vi "Process.vi"(8 "error in":errorcluster, 11 "Plugin in":refnum<class "Spectrogram.lvclass">) -> (0 "error out":errorcluster, 3 "Plugin out":refnum<class "Spectrogram.lvclass">)   [LabVIEW 2023, in "Spectrogram.lvlib" / "Spectrogram.lvclass"]
uses:
  Spectrogram.lvclass
  Spectrogram.lvclass/Spectrogram.ctl
  <vilib>/FlexLogger/SDK/PluginSDK.lvlibp/PEFClasses/SDK/Plugin/Plugin.lvclass
  C:/Program Files/National Instruments/LabVIEW 2023/vi.lib/FlexLogger/SDK/PluginSDK.lvlibp/PEFClasses/SDK/Plugin/Plugin.lvclass
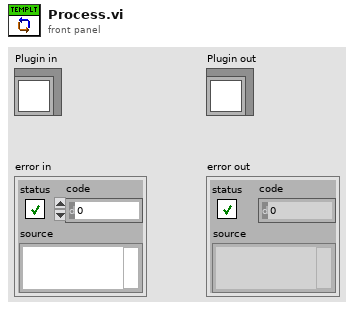
[diagram p1: front panel]
types:
  T1 = typedef "Spectrogram.lvlib/Spectrogram.lvclass/Spectrogram Data.ctl" = cluster{"First Time":bool, "Show Spectrogram Window":bool, "Show Spectrogram Window Button Clicked":bool, "Extension":u16, "Time steps":i32, "Frequency bins":i32, "Type":i32, "Length":i32, "Color Table":u16, "Spectrogram VI Ref":refnum<vi>}
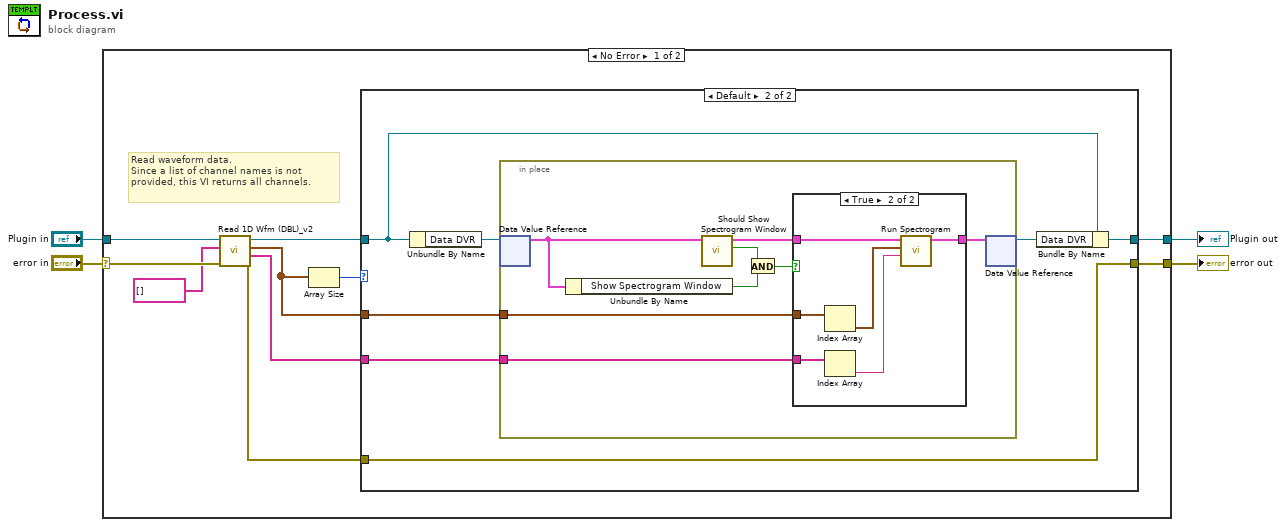
[diagram p0: block diagram]
diagram:
  n1 = case shown="No Error" "error in" {
    selector: "error in" -> [w13 w39]
    tunnel: [w11 w40] -> w1
    tunnel: "Plugin in" -> [w14 w40]
    tunnel: [w12 w39] -> w2
    frame No Error {
      # "Read waveform data.\nSince a list of channel names is not provided, this VI returns all channels."
      n2 = call <vilib>:"Read 1D Wfm (DBL)_v2.vi"("error in (no error)"=w13, "Unique Identifers (empty = all)"=string[] [] ("Unique Channel Identifers (empty = all)"), "Plugin in"=w14) -> ("error out"=w7:errorcluster, "Stream Names"=w5:string[], "Data"=w10:waveform(dbl)[], "Plugin out"=w8:refnum<class "Spectrogram.lvclass">)  [unwired: 5 in]
      n3 = Array Size(array=w10) -> (size(s)=w9:i32)
      n4 = case shown="Default" w9 {
        tunnel: w10 -> [_ w23]
        tunnel: [w15 w22] -> w12
        tunnel: [w16 w17] -> w11
        tunnel: w8 -> [w16 w18]
        tunnel: w7 -> [w15 w22]
        tunnel: w5 -> [_ w21]
        frame 0 {
          # "No channels sending data to the plugin"
        }
        frame Default {
          n5 = Unbundle By Name(w18) -> ("Data DVR"=w20:refnum<data-value>)
          n6 = in-place {
            in-place-border: w23 -> [w31]
            in-place-border: w21 -> [w28]
            n7 = in-place-dvr #1(w20) -> (w25:T1)  [unwired: 1 out]
            n8 = Unbundle By Name(w25) -> ("Show Spectrogram Window"=w30:bool)
            n9 = call "Should Show Spectrogram Window.vi"("Data in"=w25) -> ("Show Window"=w27:bool, "Data out"=w26:T1)  [unwired: 9 in]
            n10 = And(x=w27, y=w30) -> (x .and. y?=w29:bool)
            n11 = case shown="True" w29 {
              tunnel: w31 -> [_ w38]
              tunnel: w26 -> [w32 w36]
              tunnel: [w32 w35] -> w24
              tunnel: w28 -> [_ w37]
              frame False {
              }
              frame True {
                n12 = Index Array(array=w38) -> (element=w34:waveform(dbl))  [unwired: 1 in]
                n13 = Index Array(array=w37) -> (element=w33:string)  [unwired: 1 in]
                n14 = call "Run Spectrogram.vi"("Channel Name"=w33, "Signal"=w34, "Data in"=w36) -> ("Data out"=w35:T1)  [unwired: 8 in]
              }
            }
            n15 = in-place-dvr #1(w24) -> (w19:refnum<data-value>)  [unwired: 1 out]
          }
          n16 = Bundle By Name(cluster=w18, "Data DVR"=w19) -> (w17:refnum<class "Spectrogram.lvclass">)
        }
      }
    }
    frame Error {
    }
  }
  "error out" <- w2
  "Plugin out" <- w1
